vi "ChangeSIServer.vi"() -> (0 "error out":errorcluster)   [LabVIEW 2015]
uses:
  ChangeSI.ctl
  Users/Sherman/Desktop/BETA_GSCS/Systems/SystemUtil/Command.ctl
  Users/Sherman/Desktop/BETA_GSCS/Systems/SIcamera_Control/SIcamera_Globals.vi
  TCPServer/TCP_Global.vi
panel:
  in  "SI Manager Ref":refnum<vi>
  in  "Exposure Active?":bool
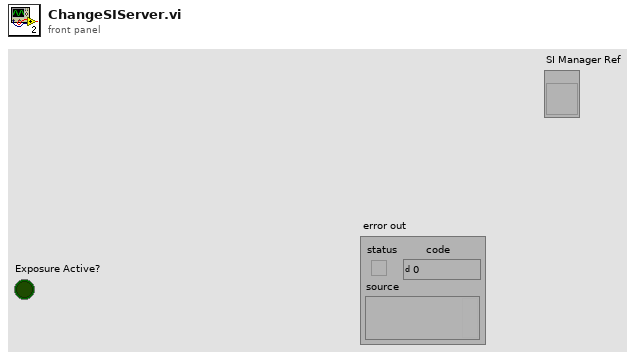
[diagram p1: front panel]
types:
  T1 = typedef "Command.ctl" = cluster{"Command":string, "Parameter":string}
  T2 = typedef "ChangeSI.ctl" = cluster{"Command":string, "SI camera info":cluster{"Observer Name":string, "object name":string, "File name base":string, "Camera Color":string, "Exp type tab":enum16{"Object", "Flat", "Comp", "Dark", "Zero", "Focus"}, "Number of Exp":i32, "Exp time":i32, "CCD Readout Speed":u8, "CCD ROI Mode":u16, "Hg(Ar)":bool, "Cu":bool, "Ne":bool, "Bulb":bool, "Ar":bool, "Quartz":bool, "Quartz Percent":i32, "Fe":bool, "Notes":string, "Target Number":string, "DomePercent":i32, "Dome":bool, "Start":dbl, "Delta":dbl, "Steps":dbl, "Custom Roi":cluster{i32, i32, i32, i32, i32, i32}}}
  T3 = cluster{"ROI Mode":refnum<vi>, "RO Speed":refnum<vi>, "File name":refnum<vi>, "Exp time":refnum<vi>, "Start exp":refnum<vi>, "num exp":refnum<vi>, "cam color":refnum<vi>, "Exp tab":refnum<vi>, "notes":refnum<vi>, "observer name":refnum<vi>, "object name":refnum<vi>, "Ar":refnum<vi>, "Bulb":refnum<vi>, "Fe":refnum<vi>, "Hg(Ar)":refnum<vi>, "Cu":refnum<vi>, "Ne":refnum<vi>, "Quartz":refnum<vi>, "Quartz percent":refnum<vi>, "flat exp":refnum<vi>, "comp exp":refnum<vi>, "dark exp":refnum<vi>, "zero exp":refnum<vi>, "Dome":refnum<vi>, "Flat Name":refnum<vi>, "Focus Name":refnum<vi>, "Focus Start":refnum<vi>, "Step Size":refnum<vi>, "Comp Name":refnum<vi>, "Comp Comments":refnum<vi>, "Focus Steps":refnum<vi>, "Dome Percent":refnum<vi>, "Dark Comments":refnum<vi>, "Zero Comments":refnum<vi>}
  T4 = cluster{"Observer Name":string, "object name":string, "File name base":string, "Camera Color":string, "Exp type tab":enum16{"Object", "Flat", "Comp", "Dark", "Zero", "Focus"}, "Number of Exp":i32, "Exp time":i32, "CCD Readout Speed":u8, "CCD ROI Mode":u16, "Hg(Ar)":bool, "Cu":bool, "Ne":bool, "Bulb":bool, "Ar":bool, "Quartz":bool, "Quartz Percent":i32, "Fe":bool, "Notes":string, "Target Number":string, "DomePercent":i32, "Dome":bool, "Start":dbl, "Delta":dbl, "Steps":dbl, "Custom Roi":cluster{i32, i32, i32, i32, i32, i32}}
  T5 = enum16{"Object", "Flat", "Comp", "Dark", "Zero", "Focus"}
  T6 = enum16{"Object", "Flat", "Comp", "Dark", "Zero", "Focus"}[]
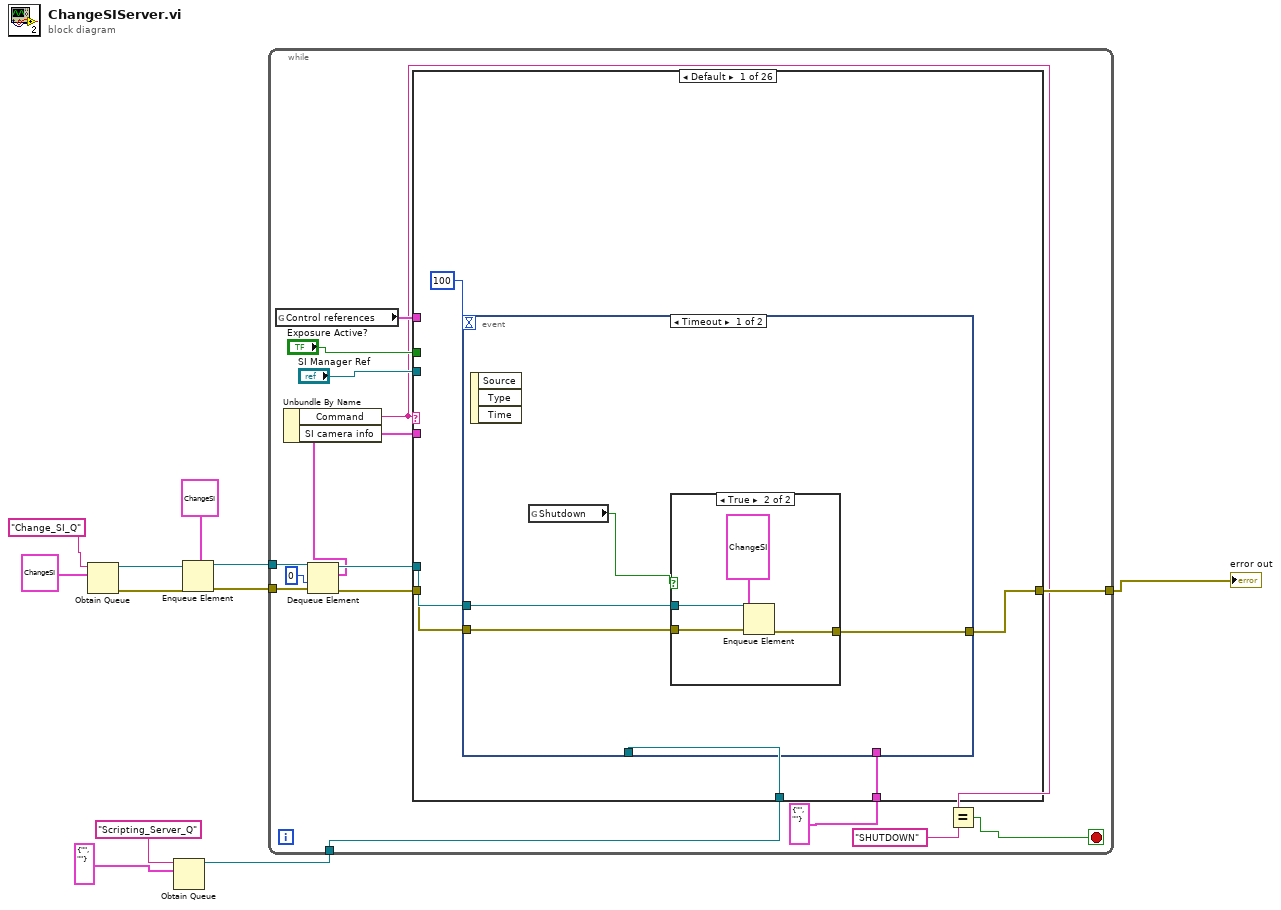
[diagram p0: block diagram]
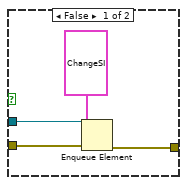
[diagram p2: hidden frame]
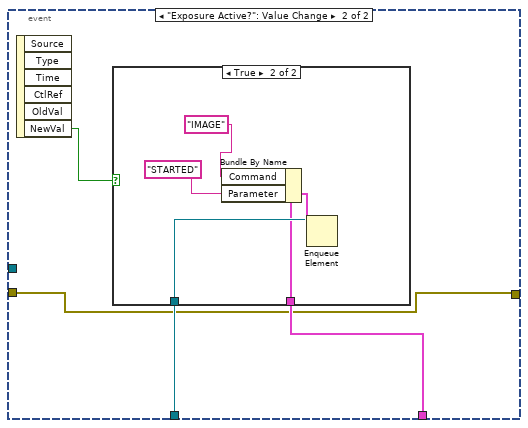
[diagram p3: hidden frame]
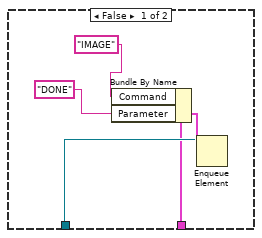
[diagram p4: hidden frame]
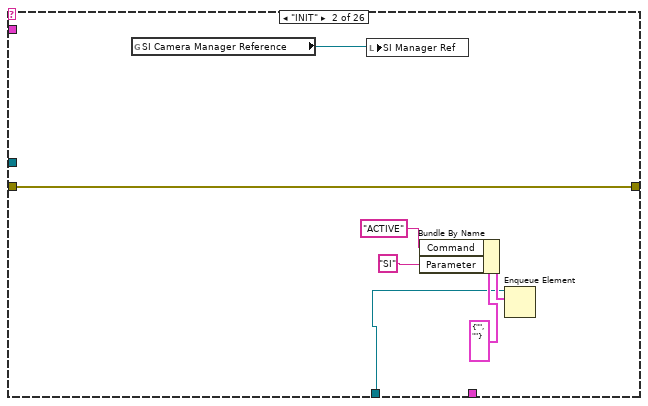
[diagram p5: hidden frame]
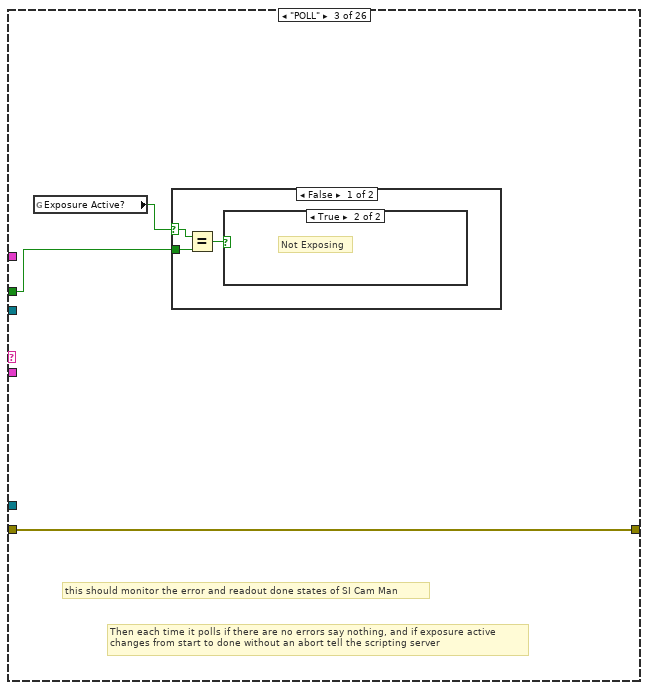
[diagram p6: hidden frame]
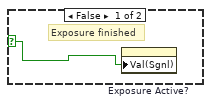
[diagram p7: hidden frame]
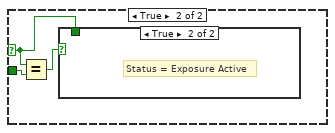
[diagram p8: hidden frame]
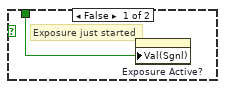
[diagram p9: hidden frame]
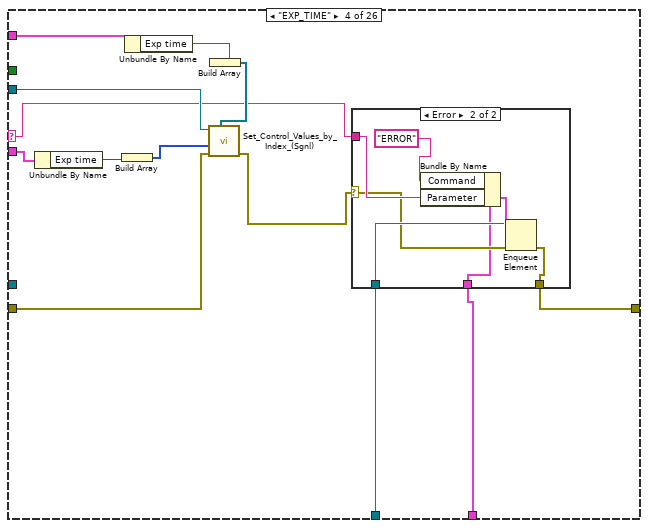
[diagram p10: hidden frame]
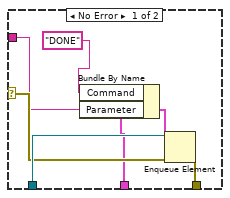
[diagram p11: hidden frame]
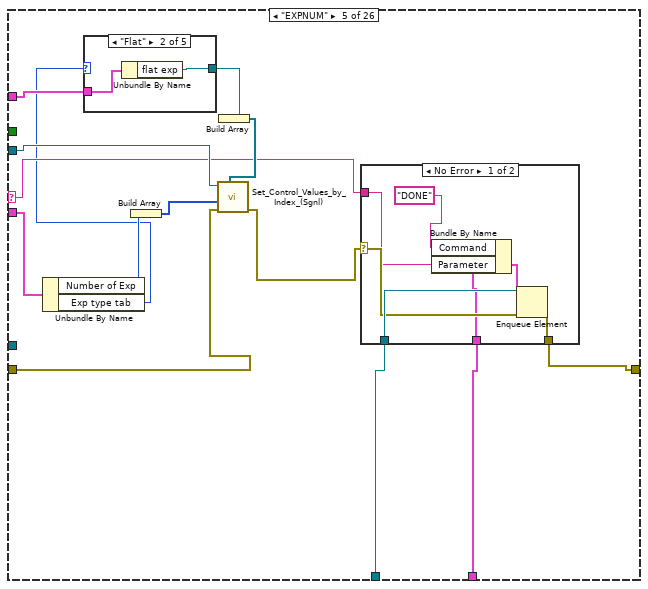
[diagram p12: hidden frame]
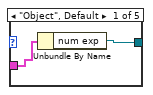
[diagram p13: hidden frame]
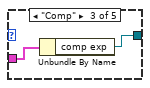
[diagram p14: hidden frame]
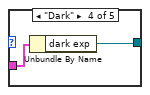
[diagram p15: hidden frame]
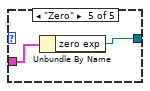
[diagram p16: hidden frame]
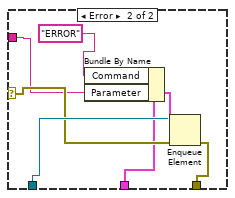
[diagram p17: hidden frame]
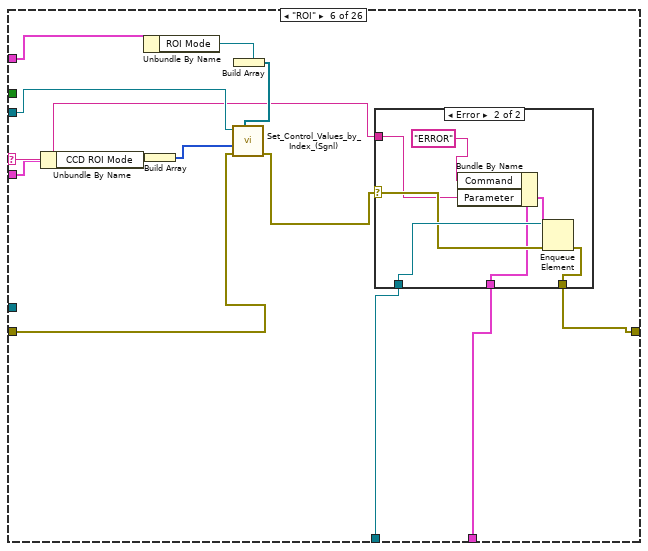
[diagram p18: hidden frame]
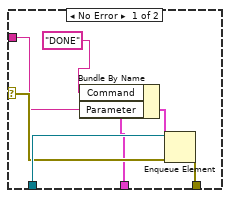
[diagram p19: hidden frame]
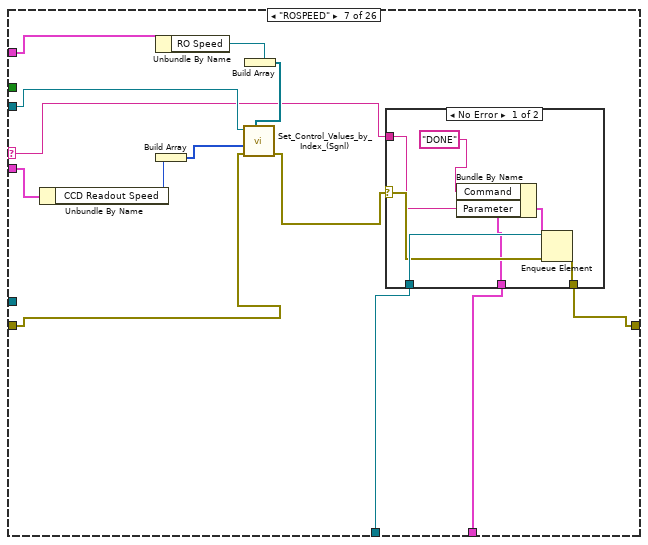
[diagram p20: hidden frame]
diagram:
  n1 = Obtain Queue(name (unnamed)="Change_SI_Q", element data type=T2 {"Command"="", "SI camera info"={"Observer Name"="", "object name"="", "File name base"="", "Camera Color"="Red", "Exp type tab"=enum."Object", "Number of Exp"=0, "Exp time"=0, "CCD Readout Speed"=5, "CCD ROI Mode"=10, "Hg(Ar)"=FALSE, "Cu"=FALSE, "Ne"=FALSE, "Bulb"=FALSE, "Ar"=FALSE, "Quartz"=FALSE, "Quartz Percent"=0, "Fe"=FALSE, "Notes"="", "Target Number"="", "DomePercent"=0, "Dome"=FALSE, "Start"=0.0, "Delta"=0.0, "Steps"=0.0, "Custom Roi"={0, 4096, 1, 0, 4096, 1}}} ("Cluster")) -> (queue out=w9:refnum<queue>, error out=w7:errorcluster)  [unwired: 3 in, 1 out]
  n2 = Obtain Queue(name (unnamed)="Scripting_Server_Q", element data type=T1 {"Command"="", "Parameter"=""} ("Command")) -> (queue out=w3:refnum<queue>)  [unwired: 3 in, 2 out]
  n3 = Enqueue Element(queue=w9, element=T2 {"Command"="INIT", "SI camera info"={"Observer Name"="", "object name"="", "File name base"="", "Camera Color"="Red", "Exp type tab"=enum."Object", "Number of Exp"=0, "Exp time"=0, "CCD Readout Speed"=5, "CCD ROI Mode"=10, "Hg(Ar)"=FALSE, "Cu"=FALSE, "Ne"=FALSE, "Bulb"=FALSE, "Ar"=FALSE, "Quartz"=FALSE, "Quartz Percent"=0, "Fe"=FALSE, "Notes"="", "Target Number"="", "DomePercent"=0, "Dome"=FALSE, "Start"=0.0, "Delta"=0.0, "Steps"=0.0, "Custom Roi"={0, 4096, 1, 0, 4096, 1}}} ("Cluster"), error in (no error)=w7) -> (queue out=w8:refnum<queue>, error out=w6:errorcluster)  [unwired: 1 in, 1 out]
  n4 = while {
    tunnel: w8 -> [w27]
    tunnel: w6 -> [w26]
    tunnel: [w20] -> w5
    tunnel: w3 -> [w19]
    stop <- w13 stop-if-true
    n5 = global read "SIcamera_Globals.vi" "Control references"() -> (w21:T3)
    n6 = Dequeue Element(queue=w27, timeout in ms (-1)=0, error in (no error)=w26) -> (queue out=w24:refnum<queue>, element=w23:T2, error out=w25:errorcluster)  [unwired: 1 out]
    n7 = Unbundle By Name(w23) -> ("Command"=w12:string, "SI camera info"=w22:T4)
    n8 = case shown="Default" w12 {
      selector: w12 -> [_ _ _ w79 w111 w148 w175 w203 w230 w257 w284 w311 w338 w364 w391 w417 w443 w469 w495 w521 w570 w623 w728 w750 w775 _]
      tunnel: w25 -> [w32 w66 w67 w86 w109 w146 w173 w200 w228 w255 w282 w309 w336 w363 w389 w415 w441 w467 w492 w519 w569 w602 w716 w749 w774 w798]
      tunnel: w24 -> [w33 _ _ _ _ _ _ _ _ _ _ _ _ _ _ _ _ _ _ _ _ _ _ _ _ w796]
      tunnel: w22 -> [_ _ _ w85 w110 w147 w174 w202 w229 w256 w283 w310 w337 w365 w390 w416 w442 w468 w494 w520 w553 w624 w729 _ _ _]
      tunnel: w21 -> [_ _ _ w89 w113 w150 w177 w205 w232 w259 w286 w313 w340 w366 w392 w418 w444 w470 w496 w522 w552 w625 w722 w751 w776 _]
      tunnel: "SI Manager Ref" -> [_ _ _ w90 w112 w149 w176 w204 w231 w258 w285 w312 w339 _ _ _ _ _ _ _ _ w610 w718 _ _ _]
      tunnel: [w29 w66 w67 w80 w108 w145 w172 w197 w225 w254 w279 w306 w333 w360 w386 w412 w438 w464 w490 w516 w566 w626 w730 w752 w777 w797] -> w20
      tunnel: w19 -> [w31 w60 _ w81 w107 w143 w170 w199 w227 w252 w281 w308 w335 w362 w388 w414 w440 w466 w493 w518 w568 w622 w727 w747 w772 w801]
      tunnel: T1 {"Command"="", "Parameter"=""} ("Command") -> [w30 _ _ w78 w106 w144 w171 w198 w226 w253 w280 w307 w334 w361 w387 w413 w439 w465 w491 w517 w567 w627 w731 w746 w771 w800]
      tunnel: "Exposure Active?" -> [_ _ w68 _ _ _ _ _ _ _ _ _ _ _ _ _ _ _ _ _ _ _ _ _ _ _]
      frame Default {
        n9 = event shown="[0] Timeout" {
          selector: _ -> [_ _]
          dyn-events: _ -> [_ _]
          timeout: 100 -> [_ _]
          tunnel: w33 -> [w37 _]
          tunnel: w32 -> [w36 w46]
          tunnel: w31 -> [_ w48]
          tunnel: w30 -> [_ w47]
          tunnel: [w35 w46] -> w29
          event Timeout {
            n10 = event-data() -> ()  [unwired: 1 in, 3 out]
            n11 = global read "TCP_Global.vi" "Shutdown"() -> (w34:bool)
            n12 = case shown="True" w34 {
              tunnel: w37 -> [w40 w44]
              tunnel: w36 -> [w39 w43]
              tunnel: [w38 w42] -> w35
              frame False {
                n13 = Enqueue Element(queue=w40, element=T2 {"Command"="POLL", "SI camera info"={"Observer Name"="", "object name"="", "File name base"="", "Camera Color"="Red", "Exp type tab"=enum."Object", "Number of Exp"=0, "Exp time"=0, "CCD Readout Speed"=5, "CCD ROI Mode"=10, "Hg(Ar)"=FALSE, "Cu"=FALSE, "Ne"=FALSE, "Bulb"=FALSE, "Ar"=FALSE, "Quartz"=FALSE, "Quartz Percent"=0, "Fe"=FALSE, "Notes"="", "Target Number"="", "DomePercent"=0, "Dome"=FALSE, "Start"=0.0, "Delta"=0.0, "Steps"=0.0, "Custom Roi"={0, 4096, 1, 0, 4096, 1}}} ("Cluster"), error in (no error)=w39) -> (error out=w38:errorcluster)  [unwired: 1 in, 2 out]
              }
              frame True {
                n14 = Enqueue Element(queue=w44, element=T2 {"Command"="QUIT", "SI camera info"={"Observer Name"="", "object name"="", "File name base"="", "Camera Color"="Red", "Exp type tab"=enum."Object", "Number of Exp"=0, "Exp time"=0, "CCD Readout Speed"=5, "CCD ROI Mode"=10, "Hg(Ar)"=FALSE, "Cu"=FALSE, "Ne"=FALSE, "Bulb"=FALSE, "Ar"=FALSE, "Quartz"=FALSE, "Quartz Percent"=0, "Fe"=FALSE, "Notes"="", "Target Number"="", "DomePercent"=0, "Dome"=FALSE, "Start"=0.0, "Delta"=0.0, "Steps"=0.0, "Custom Roi"={0, 4096, 1, 0, 4096, 1}}} ("Cluster"), error in (no error)=w43) -> (error out=w42:errorcluster)  [unwired: 1 in, 2 out]
              }
            }
          }
          event "Exposure Active?": Value Change {
            n15 = event-data() -> ("NewVal"=w49:bool)  [unwired: 1 in, 5 out]
            n16 = case shown="True" w49 {
              tunnel: w48 -> [w51 w56]
              tunnel: w47 -> [w50 w55]
              frame False {
                n17 = Bundle By Name(cluster=w50, "Command"="IMAGE", "Parameter"="DONE") -> (w54:T1)
                n18 = Enqueue Element(queue=w51, element=w54) -> ()  [unwired: 2 in, 3 out]
              }
              frame True {
                n19 = Bundle By Name(cluster=w55, "Command"="IMAGE", "Parameter"="STARTED") -> (w59:T1)
                n20 = Enqueue Element(queue=w56, element=w59) -> ()  [unwired: 2 in, 3 out]
              }
            }
          }
        }
      }
      frame "INIT" {
        n21 = global read "SIcamera_Globals.vi" "SI Camera Manager Reference"() -> (w65:refnum<vi>)
        n22 = local write "SI Manager Ref"(w65) -> ()
        n23 = Bundle By Name(cluster=T1 {"Command"="", "Parameter"=""} ("Command"), "Command"="ACTIVE", "Parameter"="SI") -> (w62:T1)
        n24 = Enqueue Element(queue=w60, element=w62) -> ()  [unwired: 2 in, 3 out]
      }
      frame "POLL" {
        # "Then each time it polls if there are no errors say nothing, and if exposure active \nchanges from start to done without an abort tell the scripting server"
        # "this should monitor the error and readout done states of SI Cam Man"
        n25 = global read "SIcamera_Globals.vi" "Exposure Active?"() -> (w69:bool)
        n26 = case shown="False" w69 {
          selector: w69 -> [w72 w74]
          tunnel: w68 -> [w71 w76]
          frame False {
            n27 = Equal?(x=w72, y=w71) -> (x = y?=w70:bool)
            n28 = case shown="True" w70 {
              selector: w70 -> [w73 _]
              frame False {
                # "Exposure finished"
                n29 = property on="Exposure Active?" class="Bool (strict)"("Val(Sgnl)"=w73) -> ()  [unwired: 2 in, 2 out]
              }
              frame True {
                # "Not Exposing"
              }
            }
          }
          frame True {
            n30 = Equal?(x=w74, y=w76) -> (x = y?=w75:bool)
            n31 = case shown="True" w75 {
              tunnel: w74 -> [w77 _]
              frame False {
                # "Exposure just started"
                n32 = property on="Exposure Active?" class="Bool (strict)"("Val(Sgnl)"=w77) -> ()  [unwired: 2 in, 2 out]
              }
              frame True {
                # "Status = Exposure Active"
              }
            }
          }
        }
      }
      frame "EXP_TIME" {
        n33 = Unbundle By Name(w85) -> ("Exp time"=w84:i32)
        n34 = Build Array(w84) -> (w83:i32[])
        n35 = Unbundle By Name(w89) -> ("Exp time"=w88:refnum<vi>)
        n36 = Build Array(w88) -> (w87:refnum<vi>[])
        n37 = call "Set_Control_Values_by_Index_(Sgnl).vi"("Control References"=w87, "error in (no error)"=w86, "appended array"=w83, "VI Refnum"=w90) -> ("error out"=w82:errorcluster)  [unwired: 6 in, 1 out]
        n38 = case shown="Error" w82 {
          selector: w82 -> [w96 w100]
          tunnel: w81 -> [w97 w101]
          tunnel: [w95 w99] -> w80
          tunnel: w79 -> [w94 w102]
          tunnel: w78 -> [w92 w98]
          frame No Error {
            n39 = Bundle By Name(cluster=w92, "Command"="DONE", "Parameter"=w94) -> (w93:T1)
            n40 = Enqueue Element(queue=w97, element=w93, error in (no error)=w96) -> (error out=w95:errorcluster)  [unwired: 1 in, 2 out]
          }
          frame Error {
            n41 = Bundle By Name(cluster=w98, "Command"="ERROR", "Parameter"=w102) -> (w104:T1)
            n42 = Enqueue Element(queue=w101, element=w104, error in (no error)=w100) -> (error out=w99:errorcluster)  [unwired: 1 in, 2 out]
          }
        }
      }
      frame "EXPNUM" {
        n43 = Unbundle By Name(w110) -> ("Number of Exp"=w116:i32, "Exp type tab"=w105:T5)
        n44 = case shown="\"Flat\"" w105 {
          tunnel: [w119 w122 w123 w125 w127] -> w118
          tunnel: w113 -> [w120 w121 w124 w126 w128]
          frame "Object", Default {
            n45 = Unbundle By Name(w120) -> ("num exp"=w119:refnum<vi>)
          }
          frame "Flat" {
            n46 = Unbundle By Name(w121) -> ("flat exp"=w122:refnum<vi>)
          }
          frame "Comp" {
            n47 = Unbundle By Name(w124) -> ("comp exp"=w123:refnum<vi>)
          }
          frame "Dark" {
            n48 = Unbundle By Name(w126) -> ("dark exp"=w125:refnum<vi>)
          }
          frame "Zero" {
            n49 = Unbundle By Name(w128) -> ("zero exp"=w127:refnum<vi>)
          }
        }
        n50 = Build Array(w116) -> (w115:i32[])
        n51 = Build Array(w118) -> (w117:refnum<vi>[])
        n52 = call "Set_Control_Values_by_Index_(Sgnl).vi"("Control References"=w117, "error in (no error)"=w109, "appended array"=w115, "VI Refnum"=w112) -> ("error out"=w114:errorcluster)  [unwired: 6 in, 1 out]
        n53 = case shown="No Error" w114 {
          selector: w114 -> [w134 w139]
          tunnel: w107 -> [w135 w140]
          tunnel: [w133 w136] -> w108
          tunnel: w111 -> [w132 w138]
          tunnel: w106 -> [w130 w137]
          frame No Error {
            n54 = Bundle By Name(cluster=w130, "Command"="DONE", "Parameter"=w132) -> (w131:T1)
            n55 = Enqueue Element(queue=w135, element=w131, error in (no error)=w134) -> (error out=w133:errorcluster)  [unwired: 1 in, 2 out]
          }
          frame Error {
            n56 = Bundle By Name(cluster=w137, "Command"="ERROR", "Parameter"=w138) -> (w142:T1)
            n57 = Enqueue Element(queue=w140, element=w142, error in (no error)=w139) -> (error out=w136:errorcluster)  [unwired: 1 in, 2 out]
          }
        }
      }
      frame "ROI" {
        n58 = Unbundle By Name(w147) -> ("CCD ROI Mode"=w153:u16)
        n59 = Unbundle By Name(w150) -> ("ROI Mode"=w155:refnum<vi>)
        n60 = Build Array(w153) -> (w152:u16[])
        n61 = Build Array(w155) -> (w154:refnum<vi>[])
        n62 = call "Set_Control_Values_by_Index_(Sgnl).vi"("Control References"=w154, "error in (no error)"=w146, "appended array"=w152, "VI Refnum"=w149) -> ("error out"=w151:errorcluster)  [unwired: 6 in, 1 out]
        n63 = case shown="Error" w151 {
          selector: w151 -> [w161 w166]
          tunnel: w143 -> [w162 w167]
          tunnel: [w160 w163] -> w145
          tunnel: w148 -> [w159 w165]
          tunnel: w144 -> [w157 w164]
          frame No Error {
            n64 = Bundle By Name(cluster=w157, "Command"="DONE", "Parameter"=w159) -> (w158:T1)
            n65 = Enqueue Element(queue=w162, element=w158, error in (no error)=w161) -> (error out=w160:errorcluster)  [unwired: 1 in, 2 out]
          }
          frame Error {
            n66 = Bundle By Name(cluster=w164, "Command"="ERROR", "Parameter"=w165) -> (w169:T1)
            n67 = Enqueue Element(queue=w167, element=w169, error in (no error)=w166) -> (error out=w163:errorcluster)  [unwired: 1 in, 2 out]
          }
        }
      }
      frame "ROSPEED" {
        n68 = Unbundle By Name(w174) -> ("CCD Readout Speed"=w180:u8)
        n69 = Unbundle By Name(w177) -> ("RO Speed"=w182:refnum<vi>)
        n70 = Build Array(w180) -> (w179:u8[])
        n71 = Build Array(w182) -> (w181:refnum<vi>[])
        n72 = call "Set_Control_Values_by_Index_(Sgnl).vi"("Control References"=w181, "error in (no error)"=w173, "appended array"=w179, "VI Refnum"=w176) -> ("error out"=w178:errorcluster)  [unwired: 6 in, 1 out]
        n73 = case shown="No Error" w178 {
          selector: w178 -> [w188 w193]
          tunnel: w170 -> [w189 w192]
          tunnel: [w187 w190] -> w172
          tunnel: w175 -> [w186 w194]
          tunnel: w171 -> [w184 w191]
          frame No Error {
            n74 = Bundle By Name(cluster=w184, "Command"="DONE", "Parameter"=w186) -> (w185:T1)
            n75 = Enqueue Element(queue=w189, element=w185, error in (no error)=w188) -> (error out=w187:errorcluster)  [unwired: 1 in, 2 out]
          }
          frame Error {
            n76 = Bundle By Name(cluster=w191, "Command"="ERROR", "Parameter"=w194) -> (w196:T1)
            n77 = Enqueue Element(queue=w192, element=w196, error in (no error)=w193) -> (error out=w190:errorcluster)  [unwired: 1 in, 2 out]
          }
        }
      }
      frame "ROTYPE" {
        n78 = Unbundle By Name(w202) -> ("Exp type tab"=w201:T5)
        n79 = Build Array(w201) -> (w207:T6)
        n80 = Unbundle By Name(w205) -> ("Exp tab"=w209:refnum<vi>)
        n81 = Build Array(w209) -> (w208:refnum<vi>[])
        n82 = call "Set_Control_Values_by_Index_(Sgnl).vi"("Control References"=w208, "error in (no error)"=w200, "appended array"=w207, "VI Refnum"=w204) -> ("error out"=w206:errorcluster)  [unwired: 6 in, 1 out]
        n83 = case shown="No Error" w206 {
          selector: w206 -> [w215 w220]
          tunnel: w199 -> [w216 w219]
          tunnel: [w214 w217] -> w197
          tunnel: w203 -> [w213 w221]
          tunnel: w198 -> [w211 w218]
          frame No Error {
            n84 = Bundle By Name(cluster=w211, "Command"="DONE", "Parameter"=w213) -> (w212:T1)
            n85 = Enqueue Element(queue=w216, element=w212, error in (no error)=w215) -> (error out=w214:errorcluster)  [unwired: 1 in, 2 out]
          }
          frame Error {
            n86 = Bundle By Name(cluster=w218, "Command"="ERROR", "Parameter"=w221) -> (w223:T1)
            n87 = Enqueue Element(queue=w219, element=w223, error in (no error)=w220) -> (error out=w217:errorcluster)  [unwired: 1 in, 2 out]
          }
        }
      }
      frame "CUSTOMROI" {
        n88 = Unbundle By Name(w229) -> ("CCD ROI Mode"=w235:u16, "Custom Roi"=w224:cluster{i32, i32, i32, i32, i32, i32})
        n89 = Unbundle By Name(w232) -> ("ROI Mode"=w237:refnum<vi>)
        n90 = Build Array(w235) -> (w234:u16[])
        n91 = Build Array(w237) -> (w236:refnum<vi>[])
        n92 = call "Set_Control_Values_by_Index_(Sgnl).vi"("Control References"=w236, "error in (no error)"=w228, "appended array"=w234, "VI Refnum"=w231) -> ("error out"=w233:errorcluster)  [unwired: 6 in, 1 out]
        n93 = global write "SIcamera_Globals.vi" "CCD ROI"(w224) -> ()
        n94 = case shown="Error" w233 {
          selector: w233 -> [w243 w249]
          tunnel: w227 -> [w244 w247]
          tunnel: [w242 w245] -> w225
          tunnel: w230 -> [w241 w248]
          tunnel: w226 -> [w239 w246]
          frame No Error {
            n95 = Bundle By Name(cluster=w239, "Command"="DONE", "Parameter"=w241) -> (w240:T1)
            n96 = Enqueue Element(queue=w244, element=w240, error in (no error)=w243) -> (error out=w242:errorcluster)  [unwired: 1 in, 2 out]
          }
          frame Error {
            n97 = Bundle By Name(cluster=w246, "Command"="ERROR", "Parameter"=w248) -> (w251:T1)
            n98 = Enqueue Element(queue=w247, element=w251, error in (no error)=w249) -> (error out=w245:errorcluster)  [unwired: 1 in, 2 out]
          }
        }
      }
      frame "FILENAME" {
        n99 = Unbundle By Name(w256) -> ("File name base"=w262:string)
        n100 = Unbundle By Name(w259) -> ("File name"=w264:refnum<vi>)
        n101 = Build Array(w262) -> (w261:string[])
        n102 = Build Array(w264) -> (w263:refnum<vi>[])
        n103 = call "Set_Control_Values_by_Index_(Sgnl).vi"("Control References"=w263, "error in (no error)"=w255, "appended array"=w261, "VI Refnum"=w258) -> ("error out"=w260:errorcluster)  [unwired: 6 in, 1 out]
        n104 = case shown="Error" w260 {
          selector: w260 -> [w270 w275]
          tunnel: w252 -> [w271 w276]
          tunnel: [w269 w272] -> w254
          tunnel: w257 -> [w268 w274]
          tunnel: w253 -> [w266 w273]
          frame No Error {
            n105 = Bundle By Name(cluster=w266, "Command"="DONE", "Parameter"=w268) -> (w267:T1)
            n106 = Enqueue Element(queue=w271, element=w267, error in (no error)=w270) -> (error out=w269:errorcluster)  [unwired: 1 in, 2 out]
          }
          frame Error {
            n107 = Bundle By Name(cluster=w273, "Command"="ERROR", "Parameter"=w274) -> (w278:T1)
            n108 = Enqueue Element(queue=w276, element=w278, error in (no error)=w275) -> (error out=w272:errorcluster)  [unwired: 1 in, 2 out]
          }
        }
      }
      frame "OBSNAME" {
        n109 = Unbundle By Name(w283) -> ("Observer Name"=w289:string)
        n110 = Unbundle By Name(w286) -> ("observer name"=w291:refnum<vi>)
        n111 = Build Array(w289) -> (w288:string[])
        n112 = Build Array(w291) -> (w290:refnum<vi>[])
        n113 = call "Set_Control_Values_by_Index_(Sgnl).vi"("Control References"=w290, "error in (no error)"=w282, "appended array"=w288, "VI Refnum"=w285) -> ("error out"=w287:errorcluster)  [unwired: 6 in, 1 out]
        n114 = case shown="Error" w287 {
          selector: w287 -> [w297 w302]
          tunnel: w281 -> [w298 w301]
          tunnel: [w296 w299] -> w279
          tunnel: w284 -> [w295 w303]
          tunnel: w280 -> [w293 w300]
          frame No Error {
            n115 = Bundle By Name(cluster=w293, "Command"="DONE", "Parameter"=w295) -> (w294:T1)
            n116 = Enqueue Element(queue=w298, element=w294, error in (no error)=w297) -> (error out=w296:errorcluster)  [unwired: 1 in, 2 out]
          }
          frame Error {
            n117 = Bundle By Name(cluster=w300, "Command"="ERROR", "Parameter"=w303) -> (w305:T1)
            n118 = Enqueue Element(queue=w301, element=w305, error in (no error)=w302) -> (error out=w299:errorcluster)  [unwired: 1 in, 2 out]
          }
        }
      }
      frame "OBJNAME" {
        n119 = Unbundle By Name(w310) -> ("object name"=w316:string)
        n120 = Unbundle By Name(w313) -> ("object name"=w318:refnum<vi>)
        n121 = Build Array(w316) -> (w315:string[])
        n122 = Build Array(w318) -> (w317:refnum<vi>[])
        n123 = call "Set_Control_Values_by_Index_(Sgnl).vi"("Control References"=w317, "error in (no error)"=w309, "appended array"=w315, "VI Refnum"=w312) -> ("error out"=w314:errorcluster)  [unwired: 6 in, 1 out]
        n124 = case shown="Error" w314 {
          selector: w314 -> [w324 w329]
          tunnel: w308 -> [w325 w328]
          tunnel: [w323 w326] -> w306
          tunnel: w311 -> [w322 w330]
          tunnel: w307 -> [w320 w327]
          frame No Error {
            n125 = Bundle By Name(cluster=w320, "Command"="DONE", "Parameter"=w322) -> (w321:T1)
            n126 = Enqueue Element(queue=w325, element=w321, error in (no error)=w324) -> (error out=w323:errorcluster)  [unwired: 1 in, 2 out]
          }
          frame Error {
            n127 = Bundle By Name(cluster=w327, "Command"="ERROR", "Parameter"=w330) -> (w332:T1)
            n128 = Enqueue Element(queue=w328, element=w332, error in (no error)=w329) -> (error out=w326:errorcluster)  [unwired: 1 in, 2 out]
          }
        }
      }
      frame "NOTES" {
        n129 = Unbundle By Name(w337) -> ("Notes"=w343:string)
        n130 = Build Array(w343) -> (w342:string[])
        n131 = Unbundle By Name(w340) -> ("notes"=w345:refnum<vi>)
        n132 = Build Array(w345) -> (w344:refnum<vi>[])
        n133 = call "Set_Control_Values_by_Index_(Sgnl).vi"("Control References"=w344, "error in (no error)"=w336, "appended array"=w342, "VI Refnum"=w339) -> ("error out"=w341:errorcluster)  [unwired: 6 in, 1 out]
        n134 = case shown="Error" w341 {
          selector: w341 -> [w351 w356]
          tunnel: w335 -> [w352 w355]
          tunnel: [w350 w353] -> w333
          tunnel: w338 -> [w349 w357]
          tunnel: w334 -> [w347 w354]
          frame No Error {
            n135 = Bundle By Name(cluster=w347, "Command"="DONE", "Parameter"=w349) -> (w348:T1)
            n136 = Enqueue Element(queue=w352, element=w348, error in (no error)=w351) -> (error out=w350:errorcluster)  [unwired: 1 in, 2 out]
          }
          frame Error {
            n137 = Bundle By Name(cluster=w354, "Command"="ERROR", "Parameter"=w357) -> (w359:T1)
            n138 = Enqueue Element(queue=w355, element=w359, error in (no error)=w356) -> (error out=w353:errorcluster)  [unwired: 1 in, 2 out]
          }
        }
      }
      frame "Hg(Ar)" {
        n139 = Unbundle By Name(w365) -> ("Hg(Ar)"=w370:bool)
        n140 = Build Array(w370) -> (w369:bool[])
        n141 = Unbundle By Name(w366) -> ("Hg(Ar)"=w371:refnum<vi>)
        n142 = Build Array(w371) -> (w367:refnum<vi>[])
        n143 = call "Set_Control_Values_by_Index_(Sgnl) for Lamps.vi"("Control References"=w367, "error in (no error)"=w363, "appended array"=w369) -> ("error out"=w368:errorcluster)  [unwired: 8 in]
        n144 = case shown="No Error" w368 {
          selector: w368 -> [w377 w382]
          tunnel: w362 -> [w378 w381]
          tunnel: [w376 w379] -> w360
          tunnel: w364 -> [w375 w383]
          tunnel: w361 -> [w373 w380]
          frame No Error {
            n145 = Bundle By Name(cluster=w373, "Command"="DONE", "Parameter"=w375) -> (w374:T1)
            n146 = Enqueue Element(queue=w378, element=w374, error in (no error)=w377) -> (error out=w376:errorcluster)  [unwired: 1 in, 2 out]
          }
          frame Error {
            n147 = Bundle By Name(cluster=w380, "Command"="ERROR", "Parameter"=w383) -> (w385:T1)
            n148 = Enqueue Element(queue=w381, element=w385, error in (no error)=w382) -> (error out=w379:errorcluster)  [unwired: 1 in, 2 out]
          }
        }
      }
      frame "Cu" {
        n149 = Unbundle By Name(w390) -> ("Cu"=w396:bool)
        n150 = Build Array(w396) -> (w395:bool[])
        n151 = Unbundle By Name(w392) -> ("Cu"=w397:refnum<vi>)
        n152 = Build Array(w397) -> (w393:refnum<vi>[])
        n153 = call "Set_Control_Values_by_Index_(Sgnl) for Lamps.vi"("Control References"=w393, "error in (no error)"=w389, "appended array"=w395) -> ("error out"=w394:errorcluster)  [unwired: 8 in]
        n154 = case shown="Error" w394 {
          selector: w394 -> [w403 w408]
          tunnel: w388 -> [w404 w407]
          tunnel: [w402 w405] -> w386
          tunnel: w391 -> [w401 w409]
          tunnel: w387 -> [w399 w406]
          frame No Error {
            n155 = Bundle By Name(cluster=w399, "Command"="DONE", "Parameter"=w401) -> (w400:T1)
            n156 = Enqueue Element(queue=w404, element=w400, error in (no error)=w403) -> (error out=w402:errorcluster)  [unwired: 1 in, 2 out]
          }
          frame Error {
            n157 = Bundle By Name(cluster=w406, "Command"="ERROR", "Parameter"=w409) -> (w411:T1)
            n158 = Enqueue Element(queue=w407, element=w411, error in (no error)=w408) -> (error out=w405:errorcluster)  [unwired: 1 in, 2 out]
          }
        }
      }
      frame "Ne" {
        n159 = Unbundle By Name(w416) -> ("Ne"=w422:bool)
        n160 = Build Array(w422) -> (w421:bool[])
        n161 = Unbundle By Name(w418) -> ("Ne"=w423:refnum<vi>)
        n162 = Build Array(w423) -> (w419:refnum<vi>[])
        n163 = call "Set_Control_Values_by_Index_(Sgnl) for Lamps.vi"("Control References"=w419, "error in (no error)"=w415, "appended array"=w421) -> ("error out"=w420:errorcluster)  [unwired: 8 in]
        n164 = case shown="Error" w420 {
          selector: w420 -> [w429 w434]
          tunnel: w414 -> [w430 w433]
          tunnel: [w428 w431] -> w412
          tunnel: w417 -> [w427 w435]
          tunnel: w413 -> [w425 w432]
          frame No Error {
            n165 = Bundle By Name(cluster=w425, "Command"="DONE", "Parameter"=w427) -> (w426:T1)
            n166 = Enqueue Element(queue=w430, element=w426, error in (no error)=w429) -> (error out=w428:errorcluster)  [unwired: 1 in, 2 out]
          }
          frame Error {
            n167 = Bundle By Name(cluster=w432, "Command"="ERROR", "Parameter"=w435) -> (w437:T1)
            n168 = Enqueue Element(queue=w433, element=w437, error in (no error)=w434) -> (error out=w431:errorcluster)  [unwired: 1 in, 2 out]
          }
        }
      }
      frame "Bulb" {
        n169 = Unbundle By Name(w442) -> ("Bulb"=w448:bool)
        n170 = Build Array(w448) -> (w447:bool[])
        n171 = Unbundle By Name(w444) -> ("Bulb"=w449:refnum<vi>)
        n172 = Build Array(w449) -> (w445:refnum<vi>[])
        n173 = call "Set_Control_Values_by_Index_(Sgnl) for Lamps.vi"("Control References"=w445, "error in (no error)"=w441, "appended array"=w447) -> ("error out"=w446:errorcluster)  [unwired: 8 in]
        n174 = case shown="Error" w446 {
          selector: w446 -> [w455 w460]
          tunnel: w440 -> [w456 w459]
          tunnel: [w454 w457] -> w438
          tunnel: w443 -> [w453 w461]
          tunnel: w439 -> [w451 w458]
          frame No Error {
            n175 = Bundle By Name(cluster=w451, "Command"="DONE", "Parameter"=w453) -> (w452:T1)
            n176 = Enqueue Element(queue=w456, element=w452, error in (no error)=w455) -> (error out=w454:errorcluster)  [unwired: 1 in, 2 out]
          }
          frame Error {
            n177 = Bundle By Name(cluster=w458, "Command"="ERROR", "Parameter"=w461) -> (w463:T1)
            n178 = Enqueue Element(queue=w459, element=w463, error in (no error)=w460) -> (error out=w457:errorcluster)  [unwired: 1 in, 2 out]
          }
        }
      }
      frame "Ar" {
        n179 = Unbundle By Name(w468) -> ("Ar"=w474:bool)
        n180 = Build Array(w474) -> (w473:bool[])
        n181 = Unbundle By Name(w470) -> ("Ar"=w475:refnum<vi>)
        n182 = Build Array(w475) -> (w471:refnum<vi>[])
        n183 = call "Set_Control_Values_by_Index_(Sgnl) for Lamps.vi"("Control References"=w471, "error in (no error)"=w467, "appended array"=w473) -> ("error out"=w472:errorcluster)  [unwired: 8 in]
        n184 = case shown="Error" w472 {
          selector: w472 -> [w481 w486]
          tunnel: w466 -> [w482 w485]
          tunnel: [w480 w483] -> w464
          tunnel: w469 -> [w479 w487]
          tunnel: w465 -> [w477 w484]
          frame No Error {
            n185 = Bundle By Name(cluster=w477, "Command"="DONE", "Parameter"=w479) -> (w478:T1)
            n186 = Enqueue Element(queue=w482, element=w478, error in (no error)=w481) -> (error out=w480:errorcluster)  [unwired: 1 in, 2 out]
          }
          frame Error {
            n187 = Bundle By Name(cluster=w484, "Command"="ERROR", "Parameter"=w487) -> (w489:T1)
            n188 = Enqueue Element(queue=w485, element=w489, error in (no error)=w486) -> (error out=w483:errorcluster)  [unwired: 1 in, 2 out]
          }
        }
      }
      frame "Quartz" {
        n189 = Unbundle By Name(w494) -> ("Quartz"=w500:bool)  [unwired: 1 out]
        n190 = Unbundle By Name(w496) -> ("Quartz"=w501:refnum<vi>)  [unwired: 1 out]
        n191 = Build Array(w500) -> (w499:bool[])
        n192 = Build Array(w501) -> (w497:refnum<vi>[])
        n193 = call "Set_Control_Values_by_Index_(Sgnl) for Lamps.vi"("Control References"=w497, "error in (no error)"=w492, "appended array"=w499) -> ("error out"=w498:errorcluster)  [unwired: 8 in]
        n194 = case shown="Error" w498 {
          selector: w498 -> [w507 w512]
          tunnel: w493 -> [w508 w511]
          tunnel: [w506 w509] -> w490
          tunnel: w495 -> [w505 w513]
          tunnel: w491 -> [w503 w510]
          frame No Error {
            n195 = Bundle By Name(cluster=w503, "Command"="DONE", "Parameter"=w505) -> (w504:T1)
            n196 = Enqueue Element(queue=w508, element=w504, error in (no error)=w507) -> (error out=w506:errorcluster)  [unwired: 1 in, 2 out]
          }
          frame Error {
            n197 = Bundle By Name(cluster=w510, "Command"="ERROR", "Parameter"=w513) -> (w515:T1)
            n198 = Enqueue Element(queue=w511, element=w515, error in (no error)=w512) -> (error out=w509:errorcluster)  [unwired: 1 in, 2 out]
          }
        }
      }
      frame "Fe" {
        n199 = Unbundle By Name(w520) -> ("Fe"=w526:bool)
        n200 = Build Array(w526) -> (w525:bool[])
        n201 = Unbundle By Name(w522) -> ("Fe"=w527:refnum<vi>)
        n202 = Build Array(w527) -> (w523:refnum<vi>[])
        n203 = call "Set_Control_Values_by_Index_(Sgnl) for Lamps.vi"("Control References"=w523, "error in (no error)"=w519, "appended array"=w525) -> ("error out"=w524:errorcluster)  [unwired: 8 in]
        n204 = case shown="No Error" w524 {
          selector: w524 -> [w533 w538]
          tunnel: w518 -> [w534 w537]
          tunnel: [w532 w535] -> w516
          tunnel: w521 -> [w531 w539]
          tunnel: w517 -> [w529 w536]
          frame No Error {
            n205 = Bundle By Name(cluster=w529, "Command"="DONE", "Parameter"=w531) -> (w530:T1)
            n206 = Enqueue Element(queue=w534, element=w530, error in (no error)=w533) -> (error out=w532:errorcluster)  [unwired: 1 in, 2 out]
          }
          frame Error {
            n207 = Bundle By Name(cluster=w536, "Command"="ERROR", "Parameter"=w539) -> (w541:T1)
            n208 = Enqueue Element(queue=w537, element=w541, error in (no error)=w538) -> (error out=w535:errorcluster)  [unwired: 1 in, 2 out]
          }
        }
      }
      frame "LAMPS" {
        n209 = Unbundle By Name(w552) -> ("Quartz percent"=w551:refnum<vi>, "Dome Percent"=w543:refnum<vi>)
        n210 = Unbundle By Name(w553) -> ("Quartz Percent"=w550:i32, "DomePercent"=w542:i32)
        n211 = Unbundle By Name(w553) -> ("Hg(Ar)"=w573:bool, "Cu"=w559:bool, "Ne"=w558:bool, "Bulb"=w557:bool, "Ar"=w556:bool, "Fe"=w555:bool, "Quartz"=w554:bool, "Dome"=w545:bool)
        n212 = Unbundle By Name(w552) -> ("Hg(Ar)"=w574:refnum<vi>, "Cu"=w565:refnum<vi>, "Ne"=w564:refnum<vi>, "Bulb"=w563:refnum<vi>, "Ar"=w562:refnum<vi>, "Fe"=w561:refnum<vi>, "Quartz"=w560:refnum<vi>, "Dome"=w544:refnum<vi>)
        n213 = Build Array(w573, w559, w558, w557, w556, w555, w554, w545) -> (w572:bool[])
        n214 = Build Array(w551, w543) -> (w549:refnum<vi>[])
        n215 = Build Array(w550, w542) -> (w548:i32[])
        n216 = Build Array(w574, w565, w564, w563, w562, w561, w560, w544) -> (w571:refnum<vi>[])
        n217 = call "Set_Control_Values_by_Index_(Sgnl) for Lamps.vi"("Control References"=w571, "error in (no error)"=w569, "appended array"=w572) -> ("error out"=w547:errorcluster)  [unwired: 8 in]
        n218 = call "Set_Control_Values_by_Index_(Sgnl) for Lamps.vi"("Control References"=w549, "error in (no error)"=w547, "appended array"=w548) -> ("error out"=w546:errorcluster)  [unwired: 8 in]
        n219 = case shown="No Error" w546 {
          selector: w546 -> [w580 w585]
          tunnel: w568 -> [w581 w584]
          tunnel: [w579 w582] -> w566
          tunnel: w570 -> [w578 w586]
          tunnel: w567 -> [w576 w583]
          frame No Error {
            n220 = Bundle By Name(cluster=w576, "Command"="DONE", "Parameter"=w578) -> (w577:T1)
            n221 = Enqueue Element(queue=w581, element=w577, error in (no error)=w580) -> (error out=w579:errorcluster)  [unwired: 1 in, 2 out]
          }
          frame Error {
            n222 = Bundle By Name(cluster=w583, "Command"="ERROR", "Parameter"=w586) -> (w588:T1)
            n223 = Enqueue Element(queue=w584, element=w588, error in (no error)=w585) -> (error out=w582:errorcluster)  [unwired: 1 in, 2 out]
          }
        }
      }
      frame "CAMSET" {
        n224 = Unbundle By Name(w624) -> ("Observer Name"=w616:string, "object name"=w617:string, "File name base"=w618:string, "Notes"=w615:string, "Exp type tab"=w589:T5, "Number of Exp"=w609:i32, "CCD ROI Mode"=w608:u16, "Exp time"=w621:i32, "CCD Readout Speed"=w604:u8, "Custom Roi"=w614:cluster{i32, i32, i32, i32, i32, i32})
        n225 = case shown="\"Object\", Default" w589 {
          tunnel: w625 -> [w640 w652 w664 w676 w688 w700]
          tunnel: [w639 w651 w663 w675 w687 w699] -> w620
          tunnel: [w634 w645 w657 w669 w681 w693] -> w605
          tunnel: [w633 w644 w656 w668 w680 w692] -> w613
          tunnel: [w630 w642 w654 w666 w678 w690] -> w607
          tunnel: [w629 w641 w653 w665 w677 w689] -> w606
          frame "Object", Default {
            n226 = Unbundle By Name(w640) -> ("observer name"=w638:refnum<vi>, "object name"=w637:refnum<vi>, "File name"=w636:refnum<vi>, "notes"=w635:refnum<vi>, "Exp tab"=w633:refnum<vi>, "num exp"=w632:refnum<vi>, "ROI Mode"=w630:refnum<vi>, "Exp time"=w631:refnum<vi>, "RO Speed"=w629:refnum<vi>)
            n227 = Build Array(w632, w631) -> (w634:refnum<vi>[])
            n228 = Build Array(w638, w637, w636, w635) -> (w639:refnum<vi>[])
          }
          frame "Flat" {
            n229 = Unbundle By Name(w652) -> ("observer name"=w650:refnum<vi>, "Flat Name"=w649:refnum<vi>, "File name"=w648:refnum<vi>, "notes"=w647:refnum<vi>, "Exp tab"=w644:refnum<vi>, "flat exp"=w646:refnum<vi>, "ROI Mode"=w642:refnum<vi>, "Exp time"=w643:refnum<vi>, "RO Speed"=w641:refnum<vi>)
            n230 = Build Array(w650, w649, w648, w647) -> (w651:refnum<vi>[])
            n231 = Build Array(w646, w643) -> (w645:refnum<vi>[])
          }
          frame "Comp" {
            n232 = Unbundle By Name(w664) -> ("observer name"=w662:refnum<vi>, "Comp Name"=w661:refnum<vi>, "File name"=w660:refnum<vi>, "notes"=w659:refnum<vi>, "Exp tab"=w656:refnum<vi>, "comp exp"=w658:refnum<vi>, "ROI Mode"=w654:refnum<vi>, "Exp time"=w655:refnum<vi>, "RO Speed"=w653:refnum<vi>)
            n233 = Build Array(w662, w661, w660, w659) -> (w663:refnum<vi>[])
            n234 = Build Array(w658, w655) -> (w657:refnum<vi>[])
          }
          frame "Dark" {
            n235 = Unbundle By Name(w676) -> ("observer name"=w674:refnum<vi>, "object name"=w673:refnum<vi>, "File name"=w672:refnum<vi>, "notes"=w671:refnum<vi>, "Exp tab"=w668:refnum<vi>, "dark exp"=w670:refnum<vi>, "ROI Mode"=w666:refnum<vi>, "Exp time"=w667:refnum<vi>, "RO Speed"=w665:refnum<vi>)
            n236 = Build Array(w674, w673, w672, w671) -> (w675:refnum<vi>[])
            n237 = Build Array(w670, w667) -> (w669:refnum<vi>[])
          }
          frame "Focus" {
            n238 = Unbundle By Name(w688) -> ("observer name"=w686:refnum<vi>, "Focus Name"=w685:refnum<vi>, "File name"=w684:refnum<vi>, "notes"=w683:refnum<vi>, "Exp tab"=w680:refnum<vi>, "num exp"=w682:refnum<vi>, "ROI Mode"=w678:refnum<vi>, "Exp time"=w679:refnum<vi>, "RO Speed"=w677:refnum<vi>)
            n239 = Build Array(w686, w685, w684, w683) -> (w687:refnum<vi>[])
            n240 = Build Array(w682, w679) -> (w681:refnum<vi>[])
          }
          frame "Zero" {
            n241 = Unbundle By Name(w700) -> ("observer name"=w698:refnum<vi>, "object name"=w697:refnum<vi>, "File name"=w696:refnum<vi>, "notes"=w695:refnum<vi>, "Exp tab"=w692:refnum<vi>, "zero exp"=w694:refnum<vi>, "ROI Mode"=w690:refnum<vi>, "Exp time"=w691:refnum<vi>, "RO Speed"=w689:refnum<vi>)
            n242 = Build Array(w698, w697, w696, w695) -> (w699:refnum<vi>[])
            n243 = Build Array(w694, w691) -> (w693:refnum<vi>[])
          }
        }
        n244 = global write "SIcamera_Globals.vi" "CCD ROI"(w614) -> ()
        n245 = Build Array(w616, w617, w618, w615) -> (w628:string[])
        n246 = Build Array(w609, w621) -> (w619:i32[])
        n247 = Build Array(w608) -> (w597:u16[])
        n248 = Build Array(w604) -> (w591:u8[])
        n249 = Build Array(w606) -> (w592:refnum<vi>[])
        n250 = Build Array(w613) -> (w612:refnum<vi>[])
        n251 = Build Array(w589) -> (w611:T6)
        n252 = call "Set_Control_Values_by_Index_(Sgnl)_ExpTab.vi"("Control References"=w612, "error in (no error)"=w602, "appended array"=w611, "VI Refnum"=w610) -> ("error out"=w601:errorcluster, "VI Refnum"=w603:refnum<vi>)  [unwired: 6 in]
        n253 = Build Array(w607) -> (w600:refnum<vi>[])
        n254 = call "Set_Control_Values_by_Index_(Sgnl).vi"("Control References"=w620, "error in (no error)"=w601, "appended array"=w628, "VI Refnum"=w603) -> ("error out"=w598:errorcluster, "VI Refnum"=w599:refnum<vi>)  [unwired: 6 in]
        n255 = call "Set_Control_Values_by_Index_(Sgnl).vi"("Control References"=w600, "error in (no error)"=w598, "appended array"=w597, "VI Refnum"=w599) -> ("error out"=w596:errorcluster, "VI Refnum"=w595:refnum<vi>)  [unwired: 6 in]
        n256 = call "Set_Control_Values_by_Index_(Sgnl).vi"("Control References"=w605, "error in (no error)"=w596, "appended array"=w619, "VI Refnum"=w595) -> ("error out"=w593:errorcluster, "VI Refnum"=w594:refnum<vi>)  [unwired: 6 in]
        n257 = call "Set_Control_Values_by_Index_(Sgnl).vi"("Control References"=w592, "error in (no error)"=w593, "appended array"=w591, "VI Refnum"=w594) -> ("error out"=w590:errorcluster)  [unwired: 6 in, 1 out]
        n258 = case shown="Error" w590 {
          selector: w590 -> [w706 w710]
          tunnel: w622 -> [w707 w711]
          tunnel: [w705 w708] -> w626
          tunnel: w623 -> [w704 w712]
          tunnel: w627 -> [w703 w709]
          frame No Error {
            n259 = Bundle By Name(cluster=w703, "Command"="DONE", "Parameter"=w704) -> (w701:T1)
            n260 = Enqueue Element(queue=w707, element=w701, error in (no error)=w706) -> (error out=w705:errorcluster)  [unwired: 1 in, 2 out]
          }
          frame Error {
            n261 = Bundle By Name(cluster=w709, "Command"="ERROR", "Parameter"=w712) -> (w714:T1)
            n262 = Enqueue Element(queue=w711, element=w714, error in (no error)=w710) -> (error out=w708:errorcluster)  [unwired: 1 in, 2 out]
          }
        }
      }
      frame "FOCUS" {
        n263 = Unbundle By Name(w722) -> ("Focus Start"=w721:refnum<vi>, "Step Size"=w720:refnum<vi>, "Focus Steps"=w719:refnum<vi>)
        n264 = Unbundle By Name(w729) -> ("Start"=w726:dbl, "Delta"=w725:dbl, "Steps"=w724:dbl)
        n265 = Build Array(w721, w720, w719) -> (w717:refnum<vi>[])
        n266 = Build Array(w726, w725, w724) -> (w723:dbl[])
        n267 = call "Set_Control_Values_by_Index_(Sgnl).vi"("Control References"=w717, "error in (no error)"=w716, "appended array"=w723, "VI Refnum"=w718) -> ("error out"=w715:errorcluster)  [unwired: 6 in, 1 out]
        n268 = case shown="No Error" w715 {
          selector: w715 -> [w737 w741]
          tunnel: w727 -> [w738 w742]
          tunnel: [w736 w739] -> w730
          tunnel: w728 -> [w735 w743]
          tunnel: w731 -> [w734 w740]
          frame No Error {
            n269 = Bundle By Name(cluster=w734, "Command"="DONE", "Parameter"=w735) -> (w732:T1)
            n270 = Enqueue Element(queue=w738, element=w732, error in (no error)=w737) -> (error out=w736:errorcluster)  [unwired: 1 in, 2 out]
          }
          frame Error {
            n271 = Bundle By Name(cluster=w740, "Command"="ERROR", "Parameter"=w743) -> (w745:T1)
            n272 = Enqueue Element(queue=w742, element=w745, error in (no error)=w741) -> (error out=w739:errorcluster)  [unwired: 1 in, 2 out]
          }
        }
      }
      frame "START" {
        n273 = Build Array(TRUE) -> (w755:bool[])
        n274 = Unbundle By Name(w751) -> ("Start exp"=w756:refnum<vi>)
        n275 = Build Array(w756) -> (w753:refnum<vi>[])
        n276 = call "Set_Control_Values_by_Index_(Sgnl) for Lamps.vi"("Control References"=w753, "error in (no error)"=w749, "appended array"=w755) -> ("error out"=w754:errorcluster)  [unwired: 8 in]
        n277 = case shown="No Error" w754 {
          selector: w754 -> [w762 w767]
          tunnel: w747 -> [w763 w766]
          tunnel: [w761 w764] -> w752
          tunnel: w750 -> [w760 w768]
          tunnel: w746 -> [w758 w765]
          frame No Error {
            n278 = Bundle By Name(cluster=w758, "Command"="DONE", "Parameter"=w760) -> (w759:T1)
            n279 = Enqueue Element(queue=w763, element=w759, error in (no error)=w762) -> (error out=w761:errorcluster)  [unwired: 1 in, 2 out]
          }
          frame Error {
            n280 = Bundle By Name(cluster=w765, "Command"="ERROR", "Parameter"=w768) -> (w770:T1)
            n281 = Enqueue Element(queue=w766, element=w770, error in (no error)=w767) -> (error out=w764:errorcluster)  [unwired: 1 in, 2 out]
          }
        }
      }
      frame "ABORT" {
        n282 = Build Array(FALSE) -> (w780:bool[])
        n283 = Unbundle By Name(w776) -> ("Start exp"=w781:refnum<vi>)
        n284 = Build Array(w781) -> (w778:refnum<vi>[])
        n285 = call "Set_Control_Values_by_Index_(Sgnl) for Lamps.vi"("Control References"=w778, "error in (no error)"=w774, "appended array"=w780) -> ("error out"=w779:errorcluster)  [unwired: 8 in]
        n286 = case shown="No Error" w779 {
          selector: w779 -> [w787 w792]
          tunnel: w772 -> [w788 w791]
          tunnel: [w786 w789] -> w777
          tunnel: w775 -> [w785 w793]
          tunnel: w771 -> [w783 w790]
          frame No Error {
            n287 = Bundle By Name(cluster=w783, "Command"="DONE", "Parameter"=w785) -> (w784:T1)
            n288 = Enqueue Element(queue=w788, element=w784, error in (no error)=w787) -> (error out=w786:errorcluster)  [unwired: 1 in, 2 out]
          }
          frame Error {
            n289 = Bundle By Name(cluster=w790, "Command"="ERROR", "Parameter"=w793) -> (w795:T1)
            n290 = Enqueue Element(queue=w791, element=w795, error in (no error)=w792) -> (error out=w789:errorcluster)  [unwired: 1 in, 2 out]
          }
        }
      }
      frame "QUIT" {
        n291 = Enqueue Element(queue=w796, element=T2 {"Command"="SHUTDOWN", "SI camera info"={"Observer Name"="", "object name"="", "File name base"="", "Camera Color"="Red", "Exp type tab"=enum."Object", "Number of Exp"=0, "Exp time"=0, "CCD Readout Speed"=5, "CCD ROI Mode"=10, "Hg(Ar)"=FALSE, "Cu"=FALSE, "Ne"=FALSE, "Bulb"=FALSE, "Ar"=FALSE, "Quartz"=FALSE, "Quartz Percent"=0, "Fe"=FALSE, "Notes"="", "Target Number"="", "DomePercent"=0, "Dome"=FALSE, "Start"=0.0, "Delta"=0.0, "Steps"=0.0, "Custom Roi"={0, 4096, 1, 0, 4096, 1}}} ("Cluster"), error in (no error)=w798) -> (error out=w797:errorcluster)  [unwired: 1 in, 2 out]
        n292 = Bundle By Name(cluster=w800, "Command"="QUIT", "Parameter"="SI") -> (w804:T1)
        n293 = Enqueue Element(queue=w801, element=w804) -> ()  [unwired: 2 in, 3 out]
      }
    }
    n294 = Equal?(x=w12, y="SHUTDOWN") -> (x = y?=w13:bool)
  }
  "error out" <- w5
